vi "apply.all.display_dates.with.cover_date.vi"() -> ()   [LabVIEW 2024]
uses:
  CV_Shared_Library/CV_Shared_Library.lvlib
  <vilib>/addons/_JKI.lib/Serialization/JSON/JKI JSON Serialization.lvlib
panel:
  out "current volume":string
  out "error out":errorcluster
  out "progress":i32(slide) scale=0.0..6573.0
  in  "Volumes Path":path=path "D:/Comics/data/cv_volumes"
  in  "Issues Path":path=path "D:/Comics/data/cv_issues"
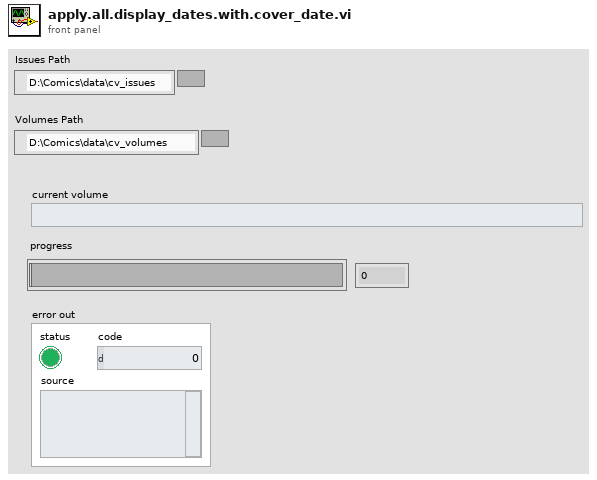
[diagram p1: front panel]
types:
  T1 = typedef "CV_RESTful_Lib.lvlib/local_issue--cluster.ctl" = cluster{"cover_date":timestamp, "id":i32, "cv_id":string, "name":string, "sortable_name":string, "issue_number":string, "deck":string, "description":string, "volume":T2, "store_date":timestamp, "date_last_updated":timestamp, "site_detail_url":string, "cover_url":string, "associated_images":T3[], "characters":T2[], "concepts":T2[], "creators":T4[], "storyArcs":T2[], "teams":T2[], "in collection":bool, "display_date":timestamp}
  T2 = typedef "CV_RESTful_Lib.lvlib/cv_issue.generic_credit--cluster.ctl" = cluster{"id":i32, "name":string}
  T3 = typedef "CV_RESTful_Lib.lvlib/cv_issue.associated_image--cluster.ctl" = cluster{"original_url":string, "id":i32}
  T4 = typedef "CV_RESTful_Lib.lvlib/cv_issue.person_credit--cluster.ctl" = cluster{"id":i32, "name":string, "role":string}
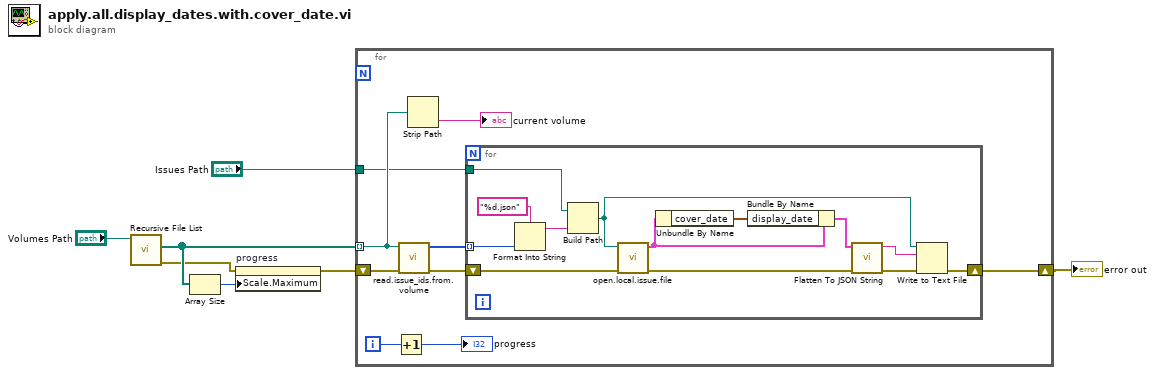
[diagram p0: block diagram]
diagram:
  n1 = call <vilib>:"Recursive File List.vi"("Folder Path"="Volumes Path") -> ("error out"=w4:errorcluster, "All Files in Dir"=w5:path[])  [unwired: 6 in, 3 out]
  n2 = Array Size(array=w5) -> (size(s)=w6:i32)
  n3 = property on="progress" class="Slide (strict)"(error in=w4, "Scale.Maximum"=w6) -> (error out=w3:errorcluster)  [unwired: 1 in, 1 out]
  n4 = for {
    tunnel: w5 -> [w11] mode=indexing
    shift-right: [w8] -> w1
    shift-left: w3 -> [w14]
    tunnel: "Issues Path" -> [w9]
    i -> [w16]
    n5 = Increment(x=w16) -> (x+1=→"progress":i32)
    n6 = call "read.issue_ids.from.volume.vi"("error in"=w14, "file (use dialog)"=w11) -> ("error out"=w12:errorcluster, "issue_ids"=w13:i32[])  [unwired: 8 in]
    n7 = Strip Path(path=w11) -> (name=→"current volume":string)  [unwired: 1 out]
    n8 = for {
      tunnel: w13 -> [w28] mode=indexing
      shift-right: [w18] -> w8
      shift-left: w12 -> [w25]
      tunnel: w9 -> [w26]
      n9 = Format Into String(format string="%d.json", w28) -> (resulting string=w27:string)  [unwired: 2 in, 1 out]
      n10 = Build Path(base path=w26, name or relative path=w27) -> (appended path=w17:path)
      n11 = call "open.local.issue.file.vi"("error in (no error)"=w25, "issue json path"=w17) -> ("error out"=w21:errorcluster, "issue"=w23:T1)  [unwired: 8 in]
      n12 = Unbundle By Name(w23) -> ("cover_date"=w24:timestamp)
      n13 = Bundle By Name(cluster=w23, "display_date"=w24) -> (w22:T1)
      n14 = call <vilib>:"Flatten To JSON String.vi"("error in"=w21, "Variant"=w22) -> ("error out"=w20:errorcluster, "JSON String"=w19:string)  [unwired: 8 in]
      n15 = Write to Text File(file (use dialog)=w17, text=w19, error in=w20) -> (error out=w18:errorcluster)  [unwired: 1 in, 2 out]
    }
  }
  "error out" <- w1
